vi "Format Arguments to JSON.vi"(1 "Arguments":string[](array[string]), 2 "Message":string) -> (0 "Output Message":string)   [LabVIEW 2019, in "TSC Event Logger.lvlib" / "JSONLayout.lvclass"]
doc: "Format the list of arguments into JSON format.\n\n<b>Code Developed By:</b>\nTechnology Service Corporation\nBloomington, IN 47403\nwww.tsc.com/atcs\n\nDeveloper:\nDaniel Coons"
uses:
  JSONLayout.lvclass
  <vilib>/Utility/error.llb/whitespace.ctl
  <vilib>/Utility/error.llb/Trim Whitespace One-Sided.vi
  <vilib>/regexp/Match Regular Expression.xnode
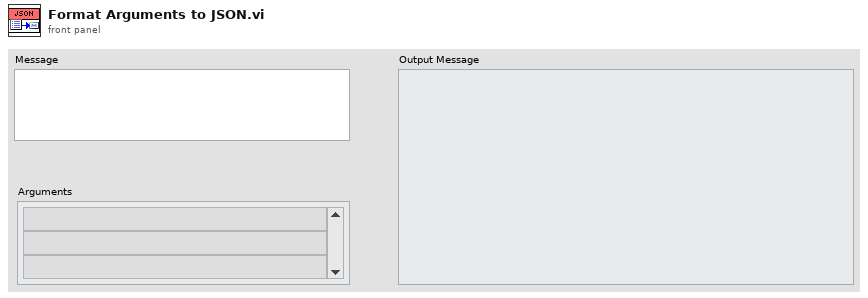
[diagram p1: front panel]
types:
  T1 = typedef "whitespace.ctl" = u16
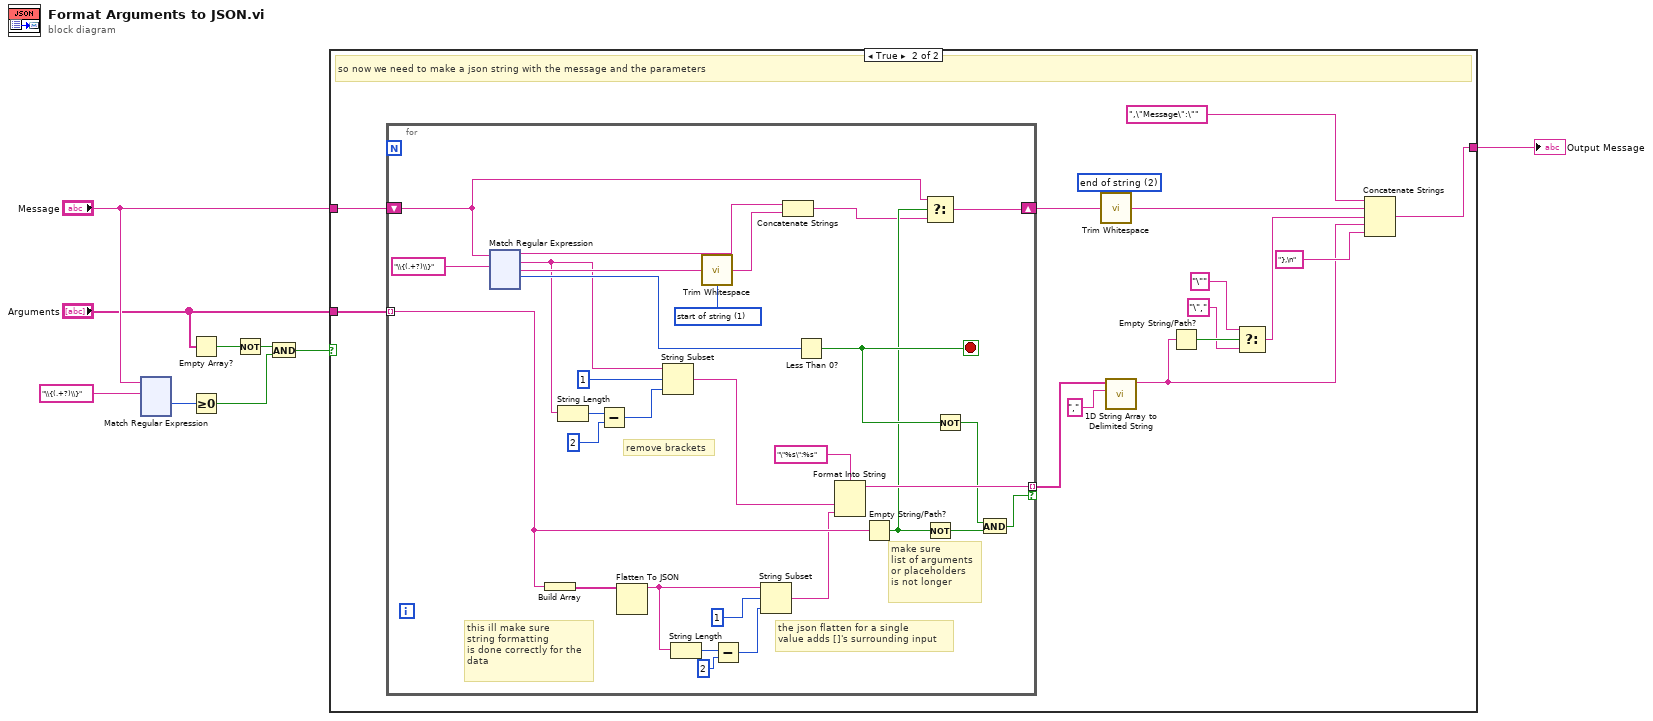
[diagram p0: block diagram]
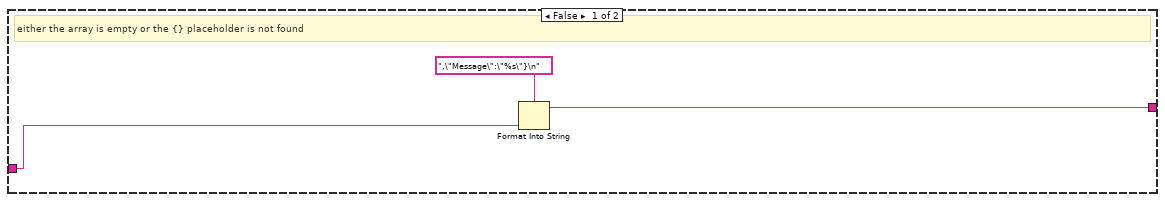
[diagram p2: hidden frame]
diagram:
  n1 = xnode "Match Regular Expression"("input string"="Message", "regular expression"="\\{(.+?)\\}") -> ("offset past match"=w7:i32)  [unwired: 4 in, 4 out]
  n2 = Empty Array?(array="Arguments") -> (empty?=w4:bool)
  n3 = Greater Or Equal To 0?(x=w7) -> (x >= 0?=w6:bool)
  n4 = Not(x=w4) -> (.not. x?=w3:bool)
  n5 = And(x=w3, y=w6) -> (x .and. y?=w2:bool)
  n6 = case shown="True" w2 {
    tunnel: "Message" -> [w11 w26]
    tunnel: "Arguments" -> [_ w27]
    tunnel: [w10 w18] -> w1
    frame False {
      # "either the array is empty or the {} placeholder is not found"
      n7 = Format Into String(format string=",\"Message\":\"%s\"}\n", w11) -> (resulting string=w10:string)  [unwired: 2 in, 1 out]
    }
    frame True {
      w22 = T1 2 items=["both", "start of string", "end of string"] ("location (both)")
      # "so now we need to make a json string with the message and the parameters"
      n8 = for {
        tunnel: w27 -> [w29] mode=indexing
        shift-right: [w37] -> w25
        shift-left: w26 -> [w36]
        tunnel: [w44] -> w24 mode=indexing if=w42
        stop <- w41 stop-if-true
        w52 = T1 1 items=["both", "start of string", "end of string"] ("location (both)")
        # "the json flatten for a single\nvalue adds []'s surrounding input"
        # "this ill make sure\nstring formatting\nis done correctly for the\ndata"
        # "make sure\nlist of arguments\nor placeholders\nis not longer"
        # "remove brackets"
        n9 = xnode "Match Regular Expression"("input string"=w36, "regular expression"="\\{(.+?)\\}") -> ("before match"=w55:string, "whole match"=w50:string, "after match"=w54:string, "offset past match"=w56:i32)  [unwired: 4 in, 1 out]
        n10 = Build Array(w29) -> (w35:string[])
        n11 = String Length(string=w50) -> (length=w49:i32)
        n12 = Subtract(x=w49, y=2) -> (x-y=w47:i32)
        n13 = Flatten To JSON(anything=w35) -> (JSON string=w33:string)  [unwired: 2 in, 1 out]
        n14 = String Subset(string=w50, offset (0)=1, length (rest)=w47) -> (substring=w45:string)
        n15 = String Length(string=w33) -> (length=w32:i32)
        n16 = call <vilib>:"Trim Whitespace.vi"("string"=w54, "location (both)"=w52) -> ("trimmed string"=w53:string)
        n17 = Subtract(x=w32, y=2) -> (x-y=w30:i32)
        n18 = String Subset(string=w33, offset (0)=1, length (rest)=w30) -> (substring=w28:string)
        n19 = Concatenate Strings(w55, w53) -> (w38:string)
        n20 = Less Than 0?(x=w56) -> (x < 0?=w41:bool)
        n21 = Format Into String(format string="\"%s\":%s", w45, w28) -> (resulting string=w44:string)  [unwired: 2 in, 1 out]
        n22 = Empty String/Path?(string/path=w29) -> (empty?=w39:bool)
        n23 = Select(t=w36, s=w39, f=w38) -> (s? t:f=w37:string)
        n24 = Not(x=w39) -> (.not. x?=w43:bool)
        n25 = Not(x=w41) -> (.not. x?=w40:bool)
        n26 = And(x=w40, y=w43) -> (x .and. y?=w42:bool)
      }
      n27 = call <vilib>:"Trim Whitespace.vi"("string"=w25, "location (both)"=w22) -> ("trimmed string"=w20:string)
      n28 = call <vilib>:"1D String Array to Delimited String.vi"("delimiter"=",", "string array"=w24) -> ("delimited string"=w17:string)  [unwired: 9 in]
      n29 = Empty String/Path?(string/path=w17) -> (empty?=w16:bool)
      n30 = Select(t="\"" ("string"), s=w16, f="\"," ("string")) -> (s? t:f=w13:string)
      n31 = Concatenate Strings(",\"Message\":\"", w20, w13, w17, "},\n" ("string")) -> (w18:string)
    }
  }
  "Output Message" <- w1
